vi "LoggerAddHandler.vi"(8 "error in (no error)":errorcluster, 10 "Handler":refnum<class "Handler.lvclass">, 11 "LoggingActor in":refnum<class "LoggingActor.lvclass">) -> (0 "error out":errorcluster, 3 "LoggingActor out":refnum<class "LoggingActor.lvclass">)   [LabVIEW 2022 SP3, in "LoggingActor.lvlib" / "LoggingActor.lvclass"]
uses:
  LoggingActor.lvclass
  Logger/Source/Handler/Handler.lvclass
  LoggingActor.lvclass/LoggingActor.ctl
  Logger/Source/Logger/Logger.lvclass
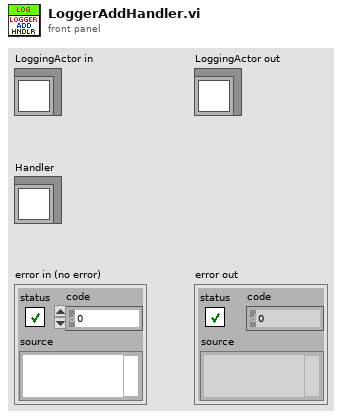
[diagram p1: front panel]
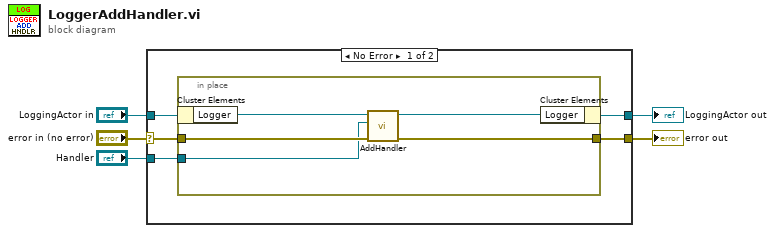
[diagram p0: block diagram]
diagram:
  n1 = case shown="No Error" "error in (no error)" {
    selector: "error in (no error)" -> [w8 w17]
    tunnel: [w7 w17] -> w4
    tunnel: [w9 w16] -> w2
    tunnel: "LoggingActor in" -> [w10 w16]
    tunnel: "Handler" -> [w6 _]
    frame No Error {
      n2 = in-place {
        in-place-border: w8 -> [w13]
        in-place-border: [w12] -> w7
        in-place-border: w6 -> [w11]
        n3 = in-place-cluster #1(w10) -> ("Logger"=w15:refnum<class "Logger.lvclass">)
        n4 = call-dynamic "AddHandler.vi"("error in (no error)"=w13, "Handler in"=w11, "Logger in"=w15) -> ("error out"=w12:errorcluster, "Logger out"=w14:refnum<class "Logger.lvclass">)  [unwired: 6 in, 1 out]
        n5 = in-place-cluster #1("Logger"=w14) -> (w9:refnum<class "LoggingActor.lvclass">)
      }
    }
    frame Error {
    }
  }
  "error out" <- w4
  "LoggingActor out" <- w2
